vi "Load Subsystem IO Alarming Attributes.vi"(7 "Headers":string[](array[string]), 8 "error in (no error)":errorcluster, 10 "Raw Configuration":string[](array[string]), 11 "Subsystem I/O Attributes In":T1={"Name"="", "Data Type"=enum."double", "Access Type"=enum."Read only", "Alarm Enabled?"=FALSE, "Logging Enabled?"=FALSE, "Logging Attributes"={"log data? (F)"=TRUE, "log alarms & events? (F)"=TRUE}, "Alarm Attributes"={"Hi:enable? (F)"=TRUE, "Hi:name"="Hi Alarm Test", "Hi:level/change"=1.0, "Lo:enable? (F)"=TRUE, "Lo:name"="Lo", "Lo:level/change"=25.0, "Boolean:enable? (F)"=TRUE, "Boolean:name"="Boolean", "Boolean:value"=TRUE, "BadStatus:enable? (F)"=TRUE, "BadStatus:name"="BadStatus"}}) -> (0 "error out":errorcluster, 2 "dup Raw Configuration":string[](array[string]), 3 "Subsystem I/O Attributes Out":T1={"Name"="", "Data Type"=enum."double", "Access Type"=enum."Read only", "Alarm Enabled?"=FALSE, "Logging Enabled?"=FALSE, "Logging Attributes"={"log data? (F)"=TRUE, "log alarms & events? (F)"=TRUE}, "Alarm Attributes"={"Hi:enable? (F)"=TRUE, "Hi:name"="Hi Alarm Test", "Hi:level/change"=1.0, "Lo:enable? (F)"=TRUE, "Lo:name"="Lo", "Lo:level/change"=25.0, "Boolean:enable? (F)"=TRUE, "Boolean:name"="Boolean", "Boolean:value"=TRUE, "BadStatus:enable? (F)"=TRUE, "BadStatus:name"="BadStatus"}})   [LabVIEW 2024]
doc: "Loads alarming attributes."
uses:
  Controls/Server/Subsystem IO Attributes.ctl
  Controls/Server/Subsystem IO Logging Attributes.ctl
  Controls/Server/Subsystem IO Alarm Attributes.ctl
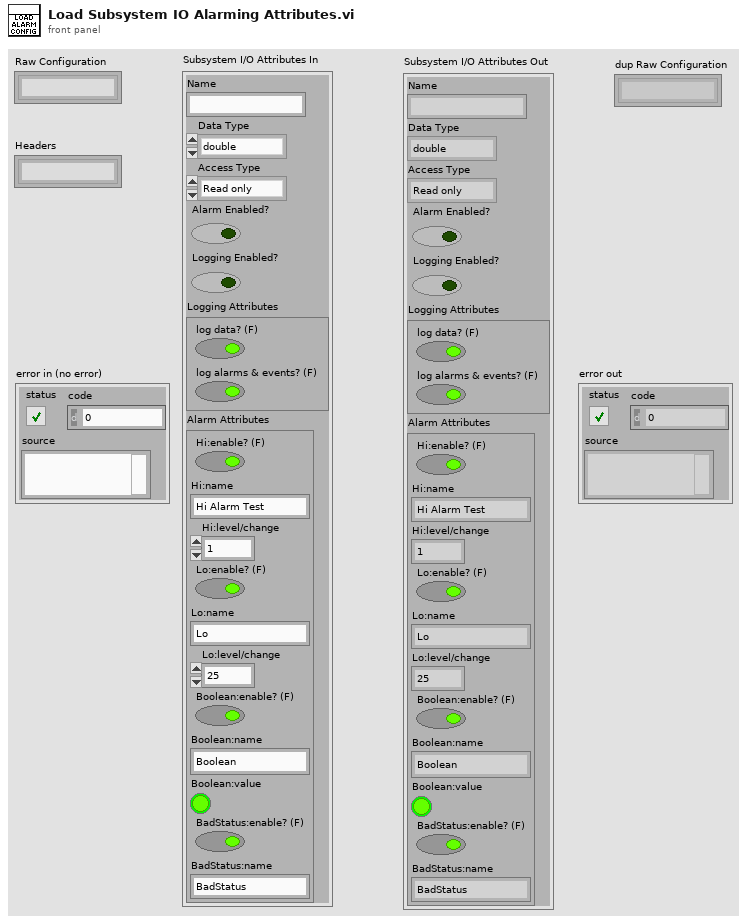
[diagram p1: front panel]
types:
  T1 = typedef "Subsystem IO Attributes.ctl" = cluster{"Name":string, "Data Type":enum32{"u32BitField", "bool", "double", "string", "int8", "uint8", "int16", "uint16", "int32", "uint32", "int64", "uint64", "single", "double waveform", "int16 waveform", "array of boolean", "array of int8", "array of uint8", "array of int16", "array of uint16", "array of int32", "array of uint32", "array of int64", "array of uint64", "array of single", "array of double", "array of double waveform", "array of int16 waveform", "array of string", "variant", "timestamp", "fixed point", "custom"}, "Access Type":enum32{"Read only", "Write only", "Read/write"}, "Alarm Enabled?":bool, "Logging Enabled?":bool, "Logging Attributes":T2, "Alarm Attributes":T3}
  T2 = typedef "Subsystem IO Logging Attributes.ctl" = cluster{"log data? (F)":bool, "log alarms & events? (F)":bool}
  T3 = typedef "Subsystem IO Alarm Attributes.ctl" = cluster{"Hi:enable? (F)":bool, "Hi:name":string, "Hi:level/change":dbl, "Lo:enable? (F)":bool, "Lo:name":string, "Lo:level/change":dbl, "Boolean:enable? (F)":bool, "Boolean:name":string, "Boolean:value":bool, "BadStatus:enable? (F)":bool, "BadStatus:name":string}
  T4 = enum32{"u32BitField", "bool", "double", "string", "int8", "uint8", "int16", "uint16", "int32", "uint32", "int64", "uint64", "single", "double waveform", "int16 waveform", "array of boolean", "array of int8", "array of uint8", "array of int16", "array of uint16", "array of int32", "array of uint32", "array of int64", "array of uint64", "array of single", "array of double", "array of double waveform", "array of int16 waveform", "array of string", "variant", "timestamp", "fixed point", "custom"}
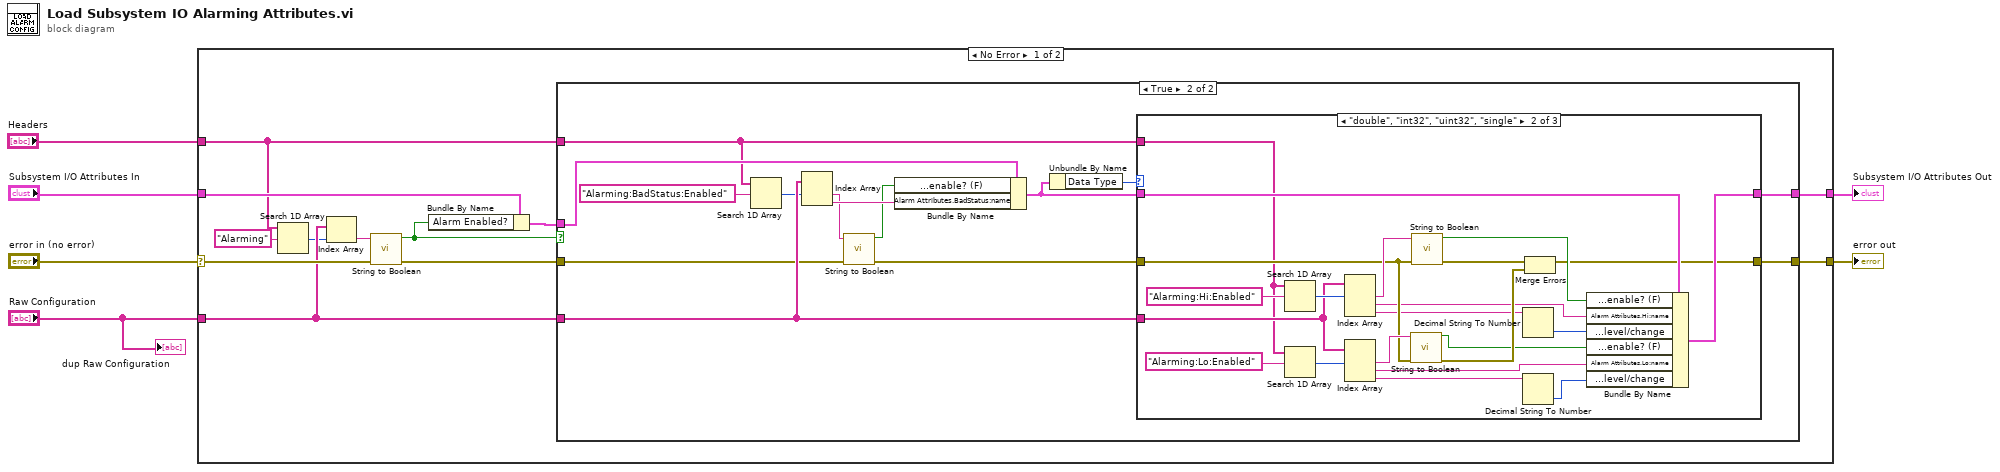
[diagram p0: block diagram]
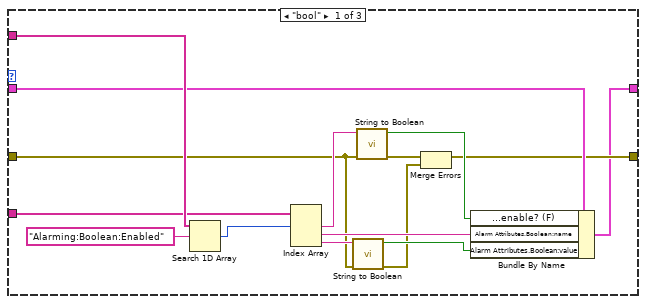
[diagram p3: hidden frame]
diagram:
  n1 = case shown="No Error" "error in (no error)" {
    selector: "error in (no error)" -> [w17 w75]
    tunnel: [w13 w75] -> w5
    tunnel: "Subsystem I/O Attributes In" -> [w12 w74]
    tunnel: [w15 w74] -> w3
    tunnel: "Raw Configuration" -> [w10 _]
    tunnel: "Headers" -> [w7 _]
    frame No Error {
      n2 = Search 1D Array(1D array=w7, element="Alarming") -> (index of element=w8:i32)  [unwired: 1 in]
      n3 = Index Array(array=w10, index=w8) -> (element=w18:string)
      n4 = call "String to Boolean.vi"("error in (no error)"=w17, "Boolean String"=w18) -> ("error out"=w14:errorcluster, "Boolean"=w11:bool)  [unwired: 8 in]
      n5 = Bundle By Name(cluster=w12, "Alarm Enabled?"=w11) -> (w16:T1)
      n6 = case shown="True" w11 {
        tunnel: w16 -> [w20 w31]
        tunnel: [w20 w23] -> w15
        tunnel: w14 -> [w19 w27]
        tunnel: [w19 w22] -> w13
        tunnel: w10 -> [_ w33]
        tunnel: w7 -> [_ w21]
        frame False {
        }
        frame True {
          n7 = Search 1D Array(1D array=w21, element="Alarming:BadStatus:Enabled") -> (index of element=w32:i32)  [unwired: 1 in]
          n8 = Index Array(array=w33, index #1=w32) -> (element #1=w29:string, element #2=w30:string)  [unwired: 1 in]
          n9 = call "String to Boolean.vi"("error in (no error)"=w27, "Boolean String"=w29) -> ("error out"=w24:errorcluster, "Boolean"=w28:bool)  [unwired: 8 in]
          n10 = Bundle By Name(cluster=w31, "Alarm Attributes.BadStatus:enable? (F)"=w28, "Alarm Attributes.BadStatus:name"=w30) -> (w25:T1)
          n11 = Unbundle By Name(w25) -> ("Data Type"=w26:T4)
          n12 = case shown="\"double\", \"int32\", \"uint32\", \"single\"" w26 {
            tunnel: w33 -> [w46 w66 _]
            tunnel: w21 -> [w47 w50 _]
            tunnel: w25 -> [w37 w59 w73]
            tunnel: w24 -> [w40 w61 w72]
            tunnel: [w35 w58 w73] -> w23
            tunnel: [w36 w57 w72] -> w22
            frame "bool" {
              n13 = Search 1D Array(1D array=w47, element="Alarming:Boolean:Enabled") -> (index of element=w49:i32)  [unwired: 1 in]
              n14 = Index Array(array=w46, index #1=w49) -> (element #1=w45:string, element #2=w44:string, element #3=w43:string)  [unwired: 2 in]
              n15 = call "String to Boolean.vi"("error in (no error)"=w40, "Boolean String"=w43) -> ("error out"=w38:errorcluster, "Boolean"=w41:bool)  [unwired: 8 in]
              n16 = call "String to Boolean.vi"("error in (no error)"=w40, "Boolean String"=w45) -> ("error out"=w39:errorcluster, "Boolean"=w42:bool)  [unwired: 8 in]
              n17 = Merge Errors(w39, w38) -> (w36:errorcluster)
              n18 = Bundle By Name(cluster=w37, "Alarm Attributes.Boolean:enable? (F)"=w42, "Alarm Attributes.Boolean:name"=w44, "Alarm Attributes.Boolean:value"=w41) -> (w35:T1)
            }
            frame "double", "int32", "uint32", "single" {
              n19 = Search 1D Array(1D array=w50, element="Alarming:Hi:Enabled") -> (index of element=w70:i32)  [unwired: 1 in]
              n20 = Search 1D Array(1D array=w50, element="Alarming:Lo:Enabled") -> (index of element=w67:i32)  [unwired: 1 in]
              n21 = Index Array(array=w66, index #1=w70) -> (element #1=w65:string, element #2=w56:string, element #3=w54:string)  [unwired: 2 in]
              n22 = Index Array(array=w66, index #1=w67) -> (element #1=w63:string, element #2=w55:string, element #3=w52:string)  [unwired: 2 in]
              n23 = call "String to Boolean.vi"("error in (no error)"=w61, "Boolean String"=w63) -> ("error out"=w71:errorcluster, "Boolean"=w62:bool)  [unwired: 8 in]
              n24 = call "String to Boolean.vi"("error in (no error)"=w61, "Boolean String"=w65) -> ("error out"=w60:errorcluster, "Boolean"=w64:bool)  [unwired: 8 in]
              n25 = Decimal String To Number(string=w54) -> (number=w53:i32)  [unwired: 2 in, 1 out]
              n26 = Decimal String To Number(string=w52) -> (number=w51:i32)  [unwired: 2 in, 1 out]
              n27 = Merge Errors(w60, w71) -> (w57:errorcluster)
              n28 = Bundle By Name(cluster=w59, "Alarm Attributes.Hi:enable? (F)"=w64, "Alarm Attributes.Hi:name"=w56, "Alarm Attributes.Hi:level/change"=w53, "Alarm Attributes.Lo:enable? (F)"=w62, "Alarm Attributes.Lo:name"=w55, "Alarm Attributes.Lo:level/change"=w51) -> (w58:T1)
            }
            frame Default {
            }
          }
        }
      }
    }
    frame Error {
    }
  }
  "error out" <- w5
  "Subsystem I/O Attributes Out" <- w3
  "dup Raw Configuration" <- "Raw Configuration"
